vi "TCP Engine Device Name.vi"(8 "error in":errorcluster, 10 "Hardware Info":T1[](array[typedef]) {"Is Present?" items=["Initializing"=-2, "Unknown"=-1, "Not Present"=0, "Present"=1]}, 11 "JSON String":string) -> (0 "error out":errorcluster, 3 "Engine Name":string[](array[string]))   [LabVIEW 2024, in "TCP Engine.lvlib"]
doc: "This purpose of this VI is to get all engine names from JSON Commands. \n\n\n\nAll Rights Reserved © 2017 SyncSols"
uses:
  TCP Engine.lvlib
  Main Engine/Controls/Main Engine Hardware Info Data Cluster.ctl
  Host-DQMH/Configuration/All Interface Data.ctl
  Host-DQMH/Configuration/DO Channel's.ctl
  Host-DQMH/Configuration/Analog Input Single Channel Data--Cluster.ctl
  Host-DQMH/Configuration/Config-Channel Type.ctl
  Host-DQMH/Configuration/Channel Sub-Type.ctl
  Analog Output/Controls/AO Timing Cluster.ctl
  Async Serial/Controls/Async Serial Configuration Cluster.ctl
  Async Serial/Controls/Async Frame Info Cluster.ctl
  Async Serial/Controls/Async Message Info Cluster.ctl
  Async Serial/Controls/Async Update Cluster.ctl
  Ethernet/Controls/Ethernet Configuration Cluster.ctl
  Ethernet/Controls/Ethernet Frame Info Cluster.ctl
  Ethernet/Controls/Ethernet Message Info Cluster.ctl
  Ethernet/Controls/Ethernet Dynamic Data Cluster.ctl
  Ethernet/Controls/Ethernet Update Cluster.ctl
  <vilib>/Utility/error.llb/Error Cluster From Error Code.vi
  <userlib>/_OpenG.lib/array/array.llb/Remove Duplicates from 1D Array (String)__ogtk.vi
  <vilib>/ErrorRing/Error Ring.xnode
  <vilib>/regexp/Match Regular Expression.xnode
  <userlib>/_OpenG.lib/array/array.llb/openg_array.lvlib
  <userlib>/_OpenG.lib/string/string.llb/openg_string.lvlib
  Host-DQMH/Configuration/Configuration.lvlib
panel:
  out "concatenated string":string
  out "Data":string
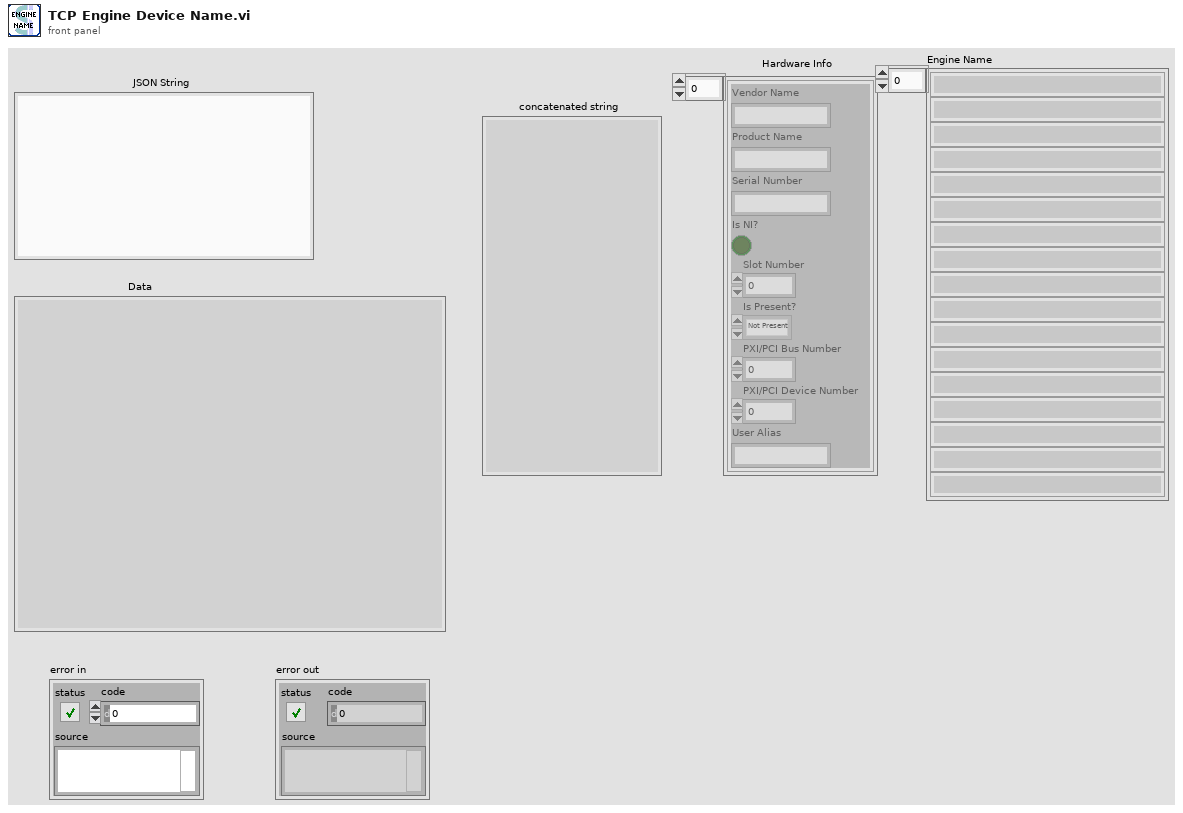
[diagram p1: front panel]
types:
  T1 = typedef "Main Engine Hardware Info Data Cluster.ctl" = cluster{"Vendor Name":string, "Product Name":string, "Serial Number":string, "Is NI?":bool, "Slot Number":i32, "Is Present?":i32, "PXI/PCI Bus Number":u32, "PXI/PCI Device Number":u32, "User Alias":string}
  T2 = typedef "Async Serial Configuration Cluster.ctl" = cluster{"Port":string, "Minor Frame Freq":u16, "Minor Frame Count":u16, "Frame Info":T3[], "Sensor Type":u16, "OIM Address":u16}
  T3 = typedef "Async Frame Info Cluster.ctl" = cluster{"Frame ID":u16, "Message Info":T4[]}
  T4 = typedef "Async Message Info Cluster.ctl" = cluster{"Message":u8[], "Message Name":string}
  T5 = typedef "Async Update Cluster.ctl" = cluster{"Port":string, "Message Info":T4[]}
  T6 = typedef "Ethernet Configuration Cluster.ctl" = cluster{"Mode":u8, "Local IP":string, "Local Port":u16, "Frame Info":T7[], "Minor Frame Freq":u8}
  T7 = typedef "Ethernet Frame Info Cluster.ctl" = cluster{"Frame ID":u16, "Message Info":T8[]}
  T8 = typedef "Ethernet Message Info Cluster.ctl" = cluster{"Message":u8[], "Message Name":string, "Dynamic":u8, "DynData":T9[], "Client IP":string, "Client Port":u16}
  T9 = typedef "Ethernet Dynamic Data Cluster.ctl" = cluster{"Type":string, "Start Byte":u8, "End Byte":u8, "Data":u32[][], "File Name":string, "Column":i32}
  T10 = typedef "Ethernet Update Cluster.ctl" = cluster{"IP":string, "Message Info":T4[], "Port":u16}
  T11 = typedef "Configuration.lvlib/All Interface Data.ctl" = cluster{"DI Config Data":T12, "DO Config Data":T12, "AI Config Data's":cluster{"Module Name":string, "AI Channel's Data":T13[], "Analog Input Timing":T16}[]}
  T12 = typedef "Configuration.lvlib/DO Channel's.ctl" = cluster{"Channel Name":string, "Identification Name":string, "Data":u8[], "Enabled?":bool}[]
  T13 = typedef "Configuration.lvlib/Analog Input Single Channel Data--Cluster.ctl" = cluster{"Channel Name":string, "Identification Name":string, "Channel Type":T14, "Sub-Type":T15, "Data":string, "Enabled?":bool}
  T14 = typedef "Configuration.lvlib/Config-Channel Type.ctl" = enum16{"Voltage", "Current", "Thermocouple", "Acclerometer"}
  T15 = typedef "Configuration.lvlib/Channel Sub-Type.ctl" = enum16{"None", "Pressure", "Force"}
  T16 = typedef "AO Timing Cluster.ctl" = cluster{"samples per channel":i32, "sample mode":i32, "Sampling Rate":dbl}
  T17 = cluster{"Module Name":string, "AI Channel's Data":T13[], "Analog Input Timing":T16}[]
  T18 = cluster{"Module Name":string, "AI Channel's Data":T13[], "Analog Input Timing":T16}
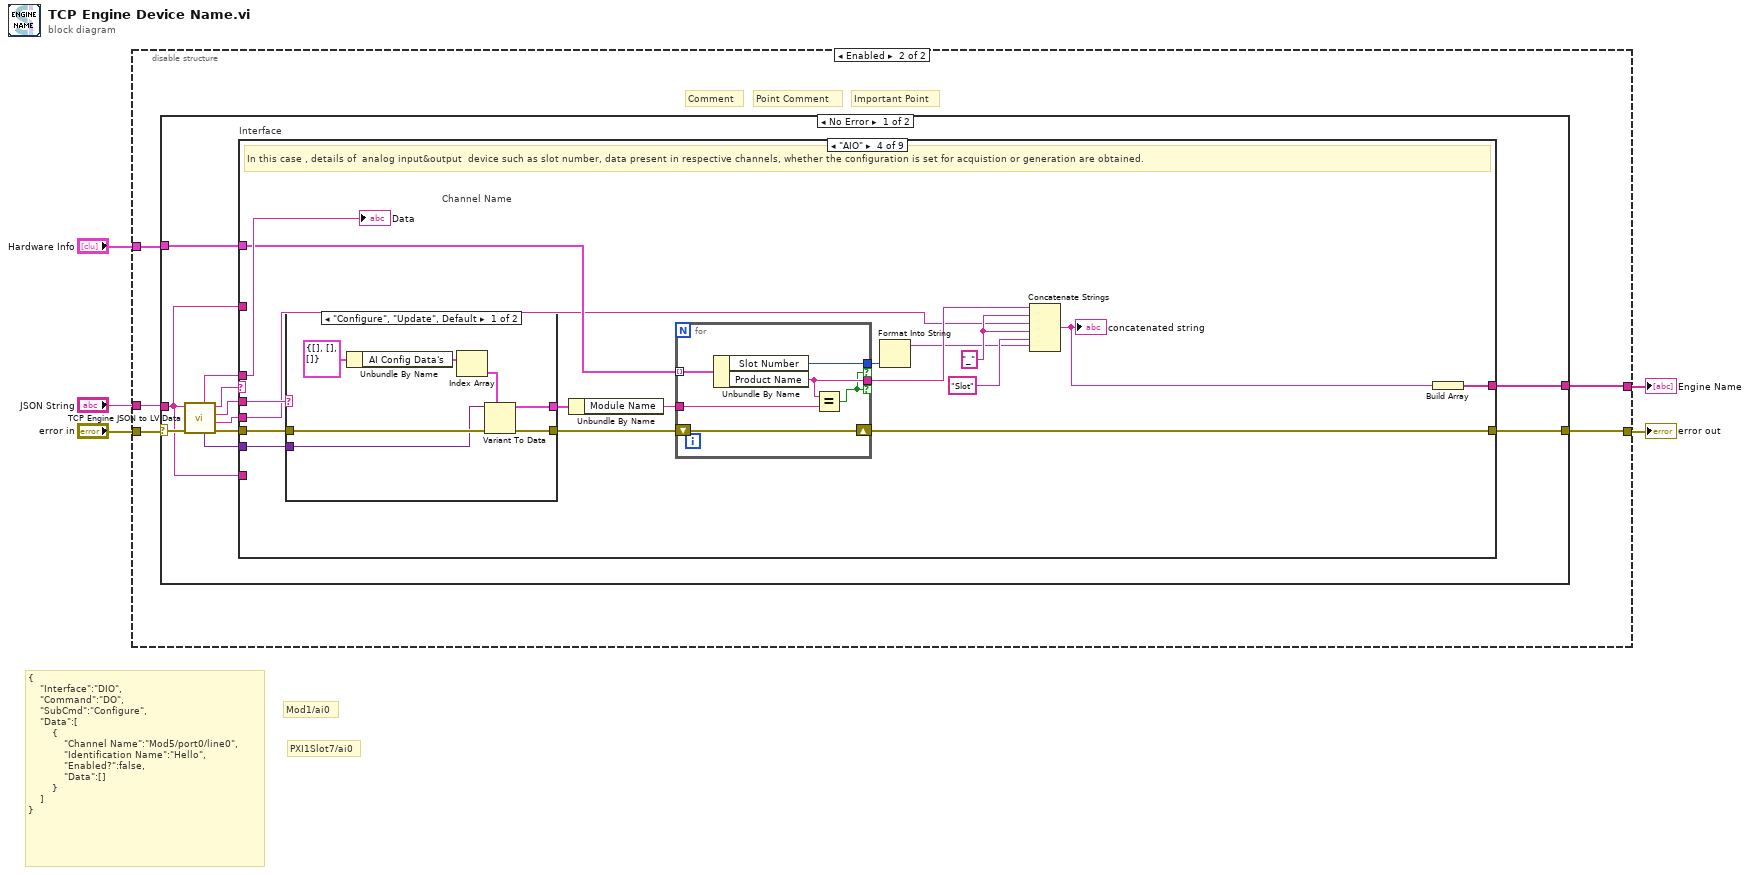
[diagram p0: block diagram]
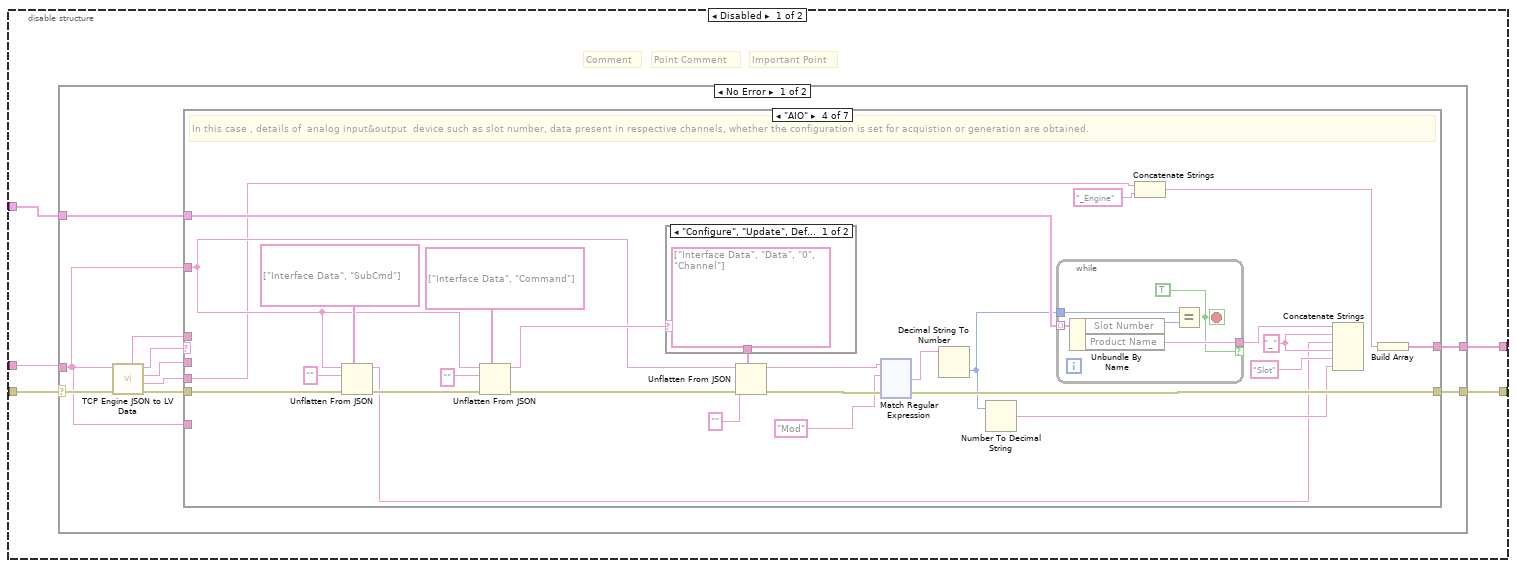
[diagram p2: hidden frame]
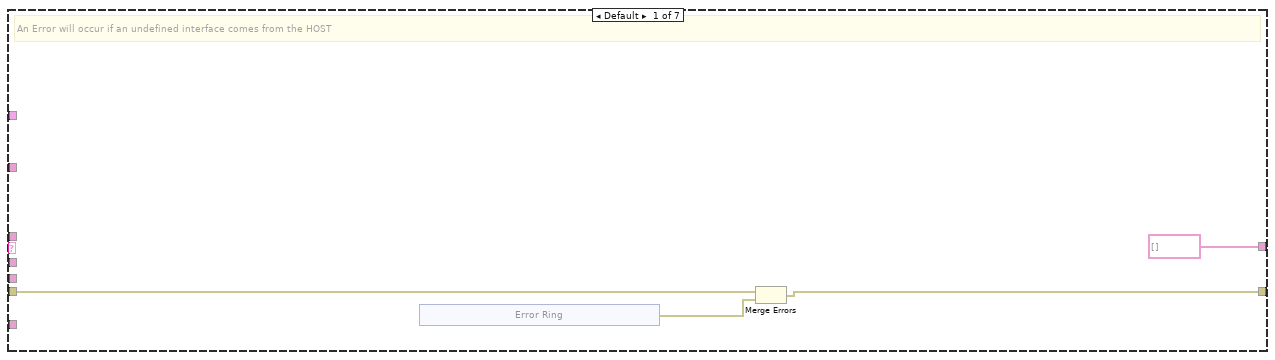
[diagram p3: hidden frame]
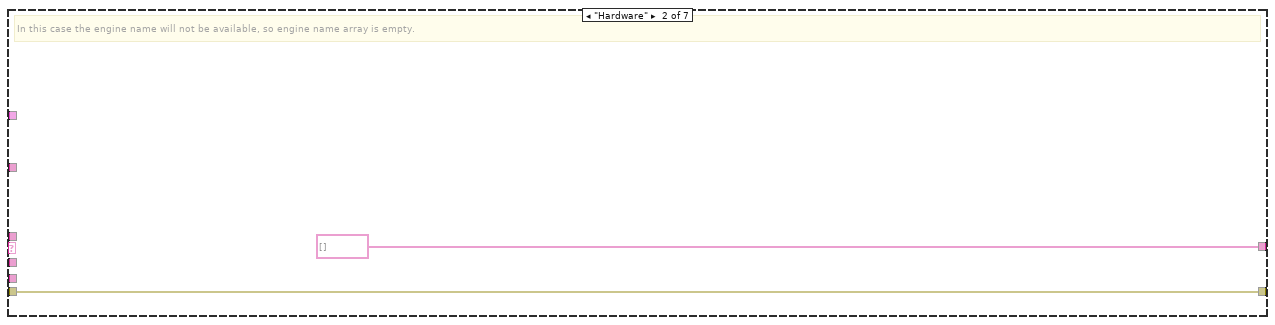
[diagram p4: hidden frame]
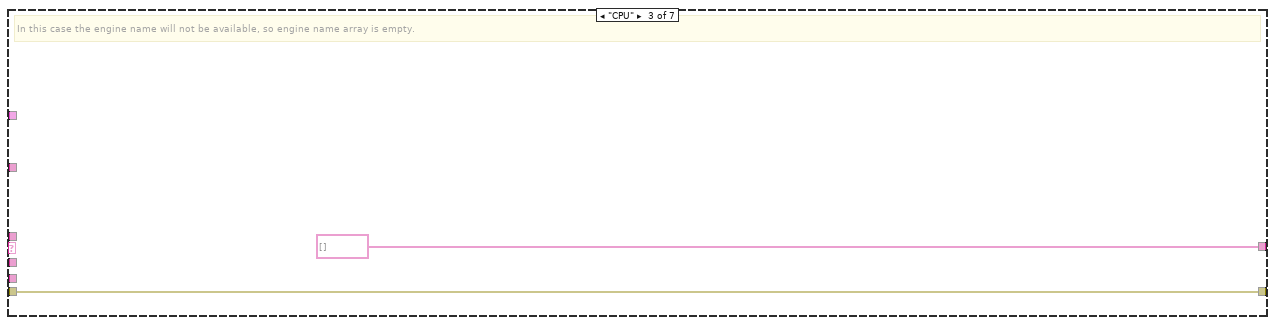
[diagram p5: hidden frame]
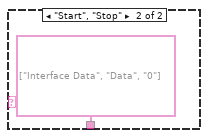
[diagram p6: hidden frame]
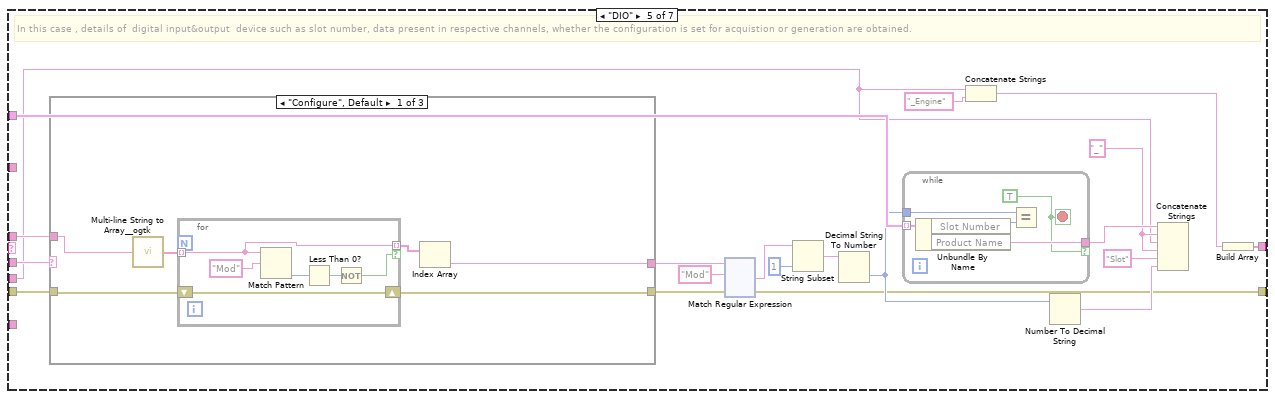
[diagram p7: hidden frame]
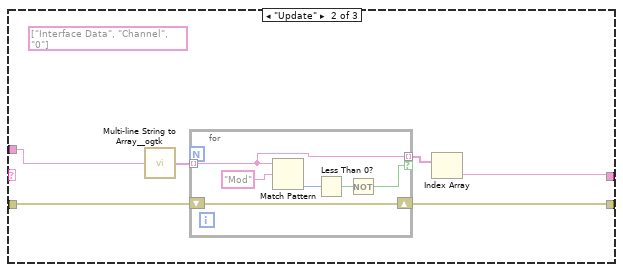
[diagram p8: hidden frame]
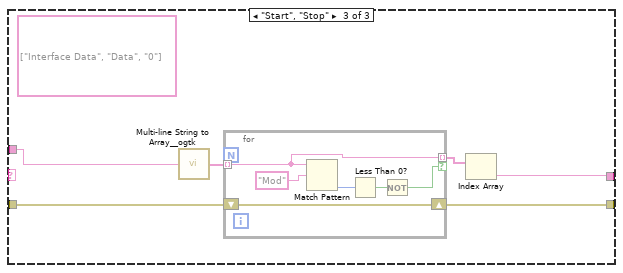
[diagram p9: hidden frame]
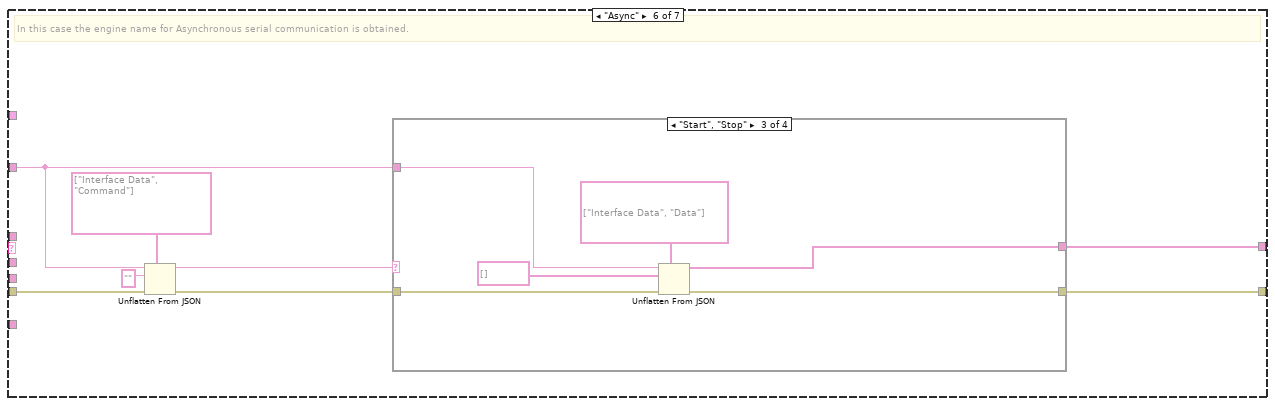
[diagram p10: hidden frame]
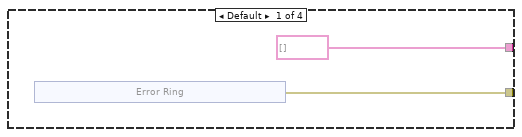
[diagram p11: hidden frame]
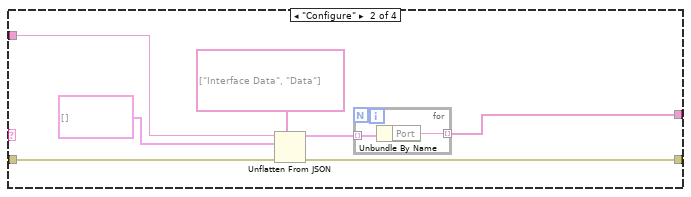
[diagram p12: hidden frame]
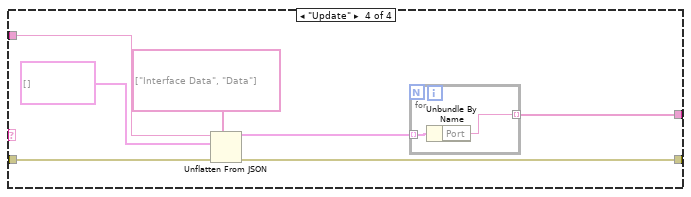
[diagram p13: hidden frame]
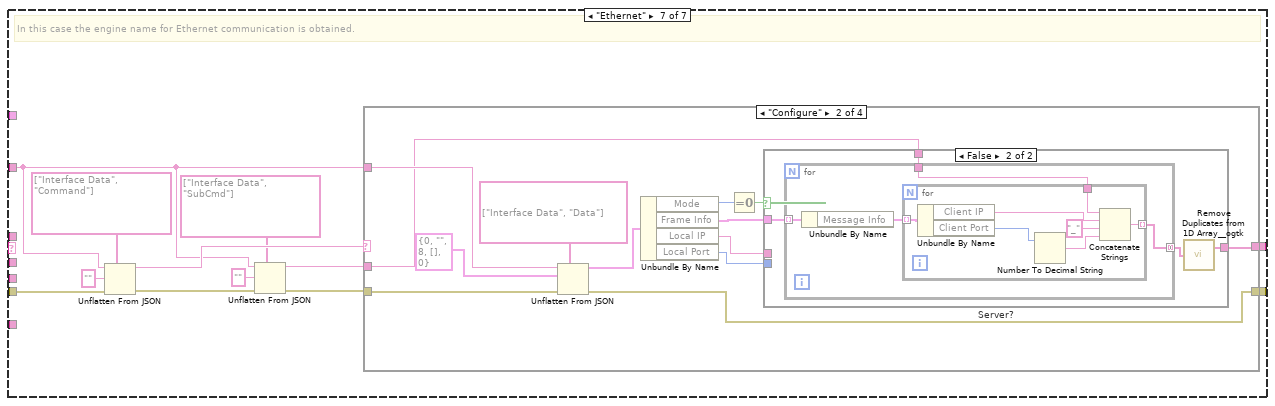
[diagram p14: hidden frame]
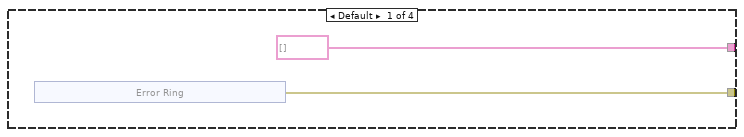
[diagram p15: hidden frame]
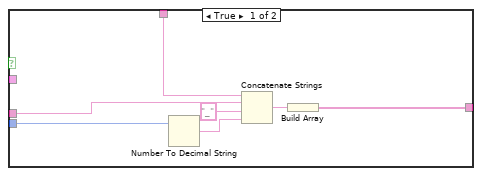
[diagram p16: hidden frame]
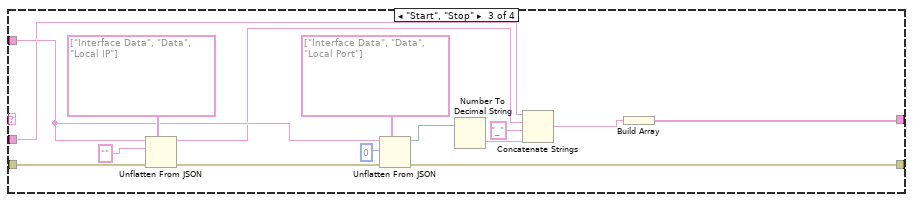
[diagram p17: hidden frame]
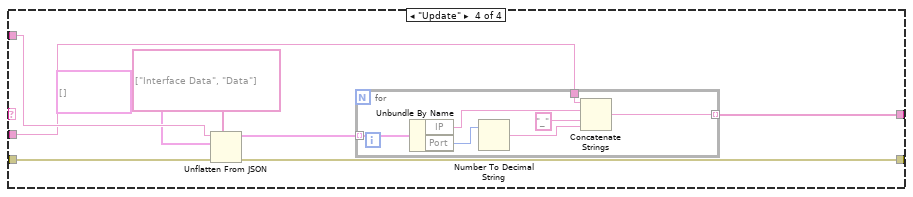
[diagram p18: hidden frame]
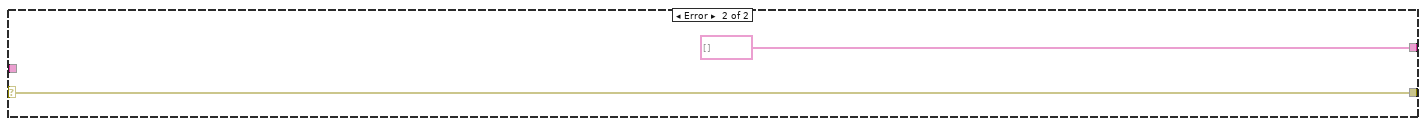
[diagram p19: hidden frame]
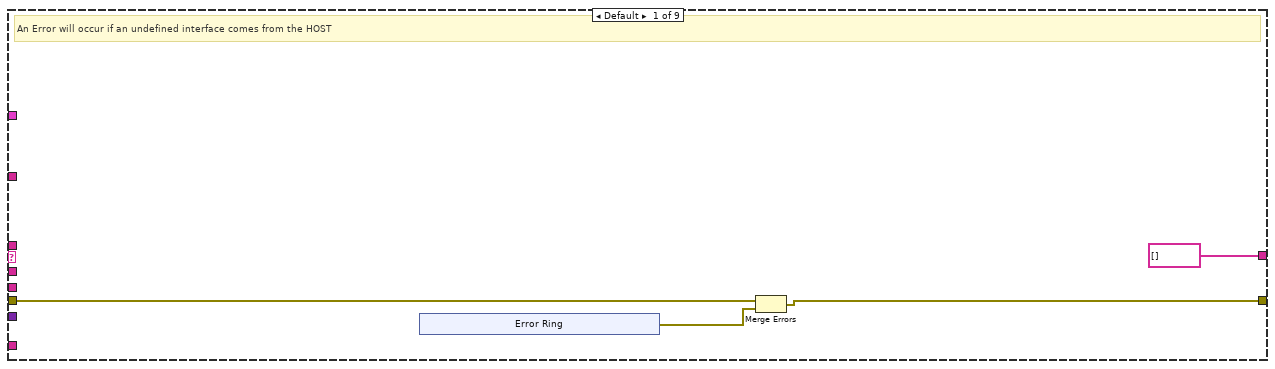
[diagram p20: hidden frame]
diagram:
  # "{\n    \"Interface\":\"DIO\",\n    \"Command\":\"DO\",\n    \"SubCmd\":\"Configure\",\n    \"Data\":[\n        {\n            \"Channel Name\":\"Mod5/port0/line0\",\n            \"Identification Name\":\"Hello\",\n            \"Enabled?\":false,\n            \"Data\":[]\n        }\n    ]\n}"
  # "Mod1/ai0"
  # "PXI1Slot7/ai0"
  n1 = disable-structure shown="Enabled" {
    disable-tunnel: "error in" -> [w10 w490]
    disable-tunnel: "JSON String" -> [w9 w491]
    disable-tunnel: "Hardware Info" -> [w8 w492]
    disable-tunnel: [w7 w488] -> w2
    disable-tunnel: [w6 w489] -> w1
    frame Disabled {
      # "Important Point"
      # "Point Comment"
      # "Comment"
      n2 = case shown="No Error" w10 {
        selector: w10 -> [w17 w487]
        tunnel: [w20 w487] -> w6
        tunnel: w9 -> [w15 _]
        tunnel: w8 -> [w19 _]
        tunnel: [w18 string[] [] ("Product Name")] -> w7
        frame No Error {
          n3 = call "TCP Engine JSON to LV Data.vi"("error in"=w17, "Cmd String"=w15) -> ("error out"=w16:errorcluster, "SubCmd"=w11:string, "Command"=w12:string, "Interface"=w14:string, "Data"=w13:string)  [unwired: 4 in, 1 out]
          n4 = case shown="\"AIO\"" w14 {
            tunnel: w15 -> [_ _ _ w37 _ w364 w403]
            tunnel: w16 -> [w21 w30 w32 w50 w198 w365 w409]
            tunnel: [w22 w30 w32 w56 w190 w370 w413] -> w20
            tunnel: w19 -> [_ _ _ w53 w204 _ _]
            tunnel: [string[] [] ("Product Name") string[] [] ("Product Name") string[] [] ("Product Name") w42 w200 w369 w412] -> w18
            tunnel: w15 -> [_ _ _ _ _ _ _]
            tunnel: w13 -> [_ _ _ _ w197 _ _]
            tunnel: w12 -> [_ _ _ _ w188 _ _]
            tunnel: w11 -> [_ _ _ w35 w187 _ _]
            frame Default {
              # "An Error will occur if an undefined interface comes from the HOST"
              n5 = xnode "Error Ring"() -> ("error out"=w24:errorcluster)
              n6 = Merge Errors(w21, w24) -> (w22:errorcluster)
            }
            frame "Hardware" {
              # "In this case the engine name will not be available, so engine name array is empty."
            }
            frame "CPU" {
              # "In this case the engine name will not be available, so engine name array is empty."
            }
            frame "AIO" {
              w41 = "_" ("string")
              # "In this case , details of  analog input&output  device such as slot number, data present in respective channels, whether the configuration is set for acquistion or generation are obtained."
              n7 = Unflatten From JSON(path=string[] ["Interface Data", "SubCmd"], JSON string=w37, type and defaults="", error in (no error)=w50) -> (value=w38:string, error out=w47:errorcluster)  [unwired: 3 in]
              n8 = Unflatten From JSON(path=string[] ["Interface Data", "Command"], JSON string=w37, type and defaults="", error in (no error)=w47) -> (value=w43:string, error out=w46:errorcluster)  [unwired: 3 in]
              n9 = case shown="\"Configure\", \"Update\", Default" w43 {
                tunnel: [string[] ["Interface Data", "Data", "0", "Channel"] ("path") string[] ["Interface Data", "Data", "0"] ("path")] -> w60
                frame "Configure", "Update", Default {
                }
                frame "Start", "Stop" {
                }
              }
              n10 = Unflatten From JSON(path=w60, JSON string=w37, type and defaults="", error in (no error)=w46) -> (value=w58:string, error out=w57:errorcluster)  [unwired: 3 in]
              n11 = xnode "Match Regular Expression"("input string"=w58, "regular expression"="Mod", "error in"=w57) -> ("after match"=w54:string, "error out"=w56:errorcluster)  [unwired: 3 in, 3 out]
              n12 = Decimal String To Number(string=w54) -> (number=w40:i32)  [unwired: 2 in, 1 out]
              n13 = Number To Decimal String(number=w40) -> (decimal integer string=w39:string)  [unwired: 1 in]
              n14 = while {
                tunnel: w53 -> [w184] mode=indexing
                tunnel: w40 -> [w182]
                tunnel: [w181] -> w52 if=w180
                stop <- w180 stop-if-true
                w180 = TRUE
                n15 = Unbundle By Name(w184) -> ("Slot Number"=w183:i32, "Product Name"=w181:string)
                n16 = Equal?(x=w182, y=w183) -> ()  [unwired: 1 out]
              }
              n17 = Concatenate Strings(w35, "_Engine" ("string")) -> (w34:string)
              n18 = Concatenate Strings(w52, w41, w38, w41, "Slot" ("string"), w39) -> ()  [unwired: 1 out]
              n19 = Build Array(w34) -> (w42:string[])
            }
            frame "DIO" {
              w201 = "_" ("string")
              # "In this case , details of  digital input&output  device such as slot number, data present in respective channels, whether the configuration is set for acquistion or generation are obtained."
              n20 = case shown="\"Configure\", Default" w188 {
                tunnel: [w323 w335 w348] -> w191
                tunnel: w198 -> [w322 w336 w349]
                tunnel: w197 -> [w325 w337 w347]
                tunnel: [w324 w334 w346] -> w189
                frame "Configure", Default {
                  n21 = call <userlib>:"Multi-line String to Array__ogtk.vi"("string"=w325) -> ("lines"=w327:string[])
                  n22 = for {
                    tunnel: w327 -> [w329] mode=indexing
                    tunnel: [w329] -> w326 mode=indexing if=w330
                    shift-right: [w328] -> w323
                    shift-left: w322 -> [w328]
                    n23 = Match Pattern(string=w329, regular expression="Mod") -> (offset past match=w332:i32)  [unwired: 1 in, 3 out]
                    n24 = Less Than 0?(x=w332) -> (x < 0?=w331:bool)
                    n25 = Not(x=w331) -> (.not. x?=w330:bool)
                  }
                  n26 = Index Array(array=w326) -> (element=w324:string)  [unwired: 1 in]
                }
                frame "Update" {
                  (unwired) string[] ["Interface Data", "Channel", "0"] ("path")
                  n27 = call <userlib>:"Multi-line String to Array__ogtk.vi"("string"=w337) -> ("lines"=w339:string[])
                  n28 = for {
                    tunnel: w339 -> [w341] mode=indexing
                    tunnel: [w341] -> w338 mode=indexing if=w342
                    shift-right: [w340] -> w335
                    shift-left: w336 -> [w340]
                    n29 = Match Pattern(string=w341, regular expression="Mod") -> (offset past match=w344:i32)  [unwired: 1 in, 3 out]
                    n30 = Less Than 0?(x=w344) -> (x < 0?=w343:bool)
                    n31 = Not(x=w343) -> (.not. x?=w342:bool)
                  }
                  n32 = Index Array(array=w338) -> (element=w334:string)  [unwired: 1 in]
                }
                frame "Start", "Stop" {
                  (unwired) string[] ["Interface Data", "Data", "0"] ("path")
                  n33 = call <userlib>:"Multi-line String to Array__ogtk.vi"("string"=w347) -> ("lines"=w351:string[])
                  n34 = for {
                    tunnel: w351 -> [w353] mode=indexing
                    tunnel: [w353] -> w350 mode=indexing if=w354
                    shift-right: [w352] -> w348
                    shift-left: w349 -> [w352]
                    n35 = Match Pattern(string=w353, regular expression="Mod") -> (offset past match=w356:i32)  [unwired: 1 in, 3 out]
                    n36 = Less Than 0?(x=w356) -> (x < 0?=w355:bool)
                    n37 = Not(x=w355) -> (.not. x?=w354:bool)
                  }
                  n38 = Index Array(array=w350) -> (element=w346:string)  [unwired: 1 in]
                }
              }
              n39 = xnode "Match Regular Expression"("input string"=w189, "regular expression"="Mod", "error in"=w191) -> ("after match"=w195:string, "error out"=w190:errorcluster)  [unwired: 3 in, 3 out]
              n40 = String Subset(string=w195, length (rest)=1 ("length (rest)")) -> (substring=w193:string)  [unwired: 1 in]
              n41 = Decimal String To Number(string=w193) -> (number=w192:i32)  [unwired: 2 in, 1 out]
              n42 = while {
                tunnel: w204 -> [w362] mode=indexing
                tunnel: w192 -> [w360]
                tunnel: [w359] -> w203 if=w358
                stop <- w358 stop-if-true
                w358 = TRUE
                n43 = Unbundle By Name(w362) -> ("Slot Number"=w361:i32, "Product Name"=w359:string)
                n44 = Equal?(x=w360, y=w361) -> ()  [unwired: 1 out]
              }
              n45 = Concatenate Strings(w187, "_Engine" ("string")) -> (w185:string)
              n46 = Number To Decimal String(number=w192) -> (decimal integer string=w199:string)  [unwired: 1 in]
              n47 = Concatenate Strings(w203, w201, w187, w201, "Slot" ("string"), w199) -> ()  [unwired: 1 out]
              n48 = Build Array(w185) -> (w200:string[])
            }
            frame "Async" {
              # "In this case the engine name for Asynchronous serial communication is obtained."
              n49 = Unflatten From JSON(path=string[] ["Interface Data", "Command"], JSON string=w364, type and defaults="", error in (no error)=w365) -> (value=w363:string, error out=w366:errorcluster)  [unwired: 3 in]
              n50 = case shown="\"Start\", \"Stop\"" w363 {
                tunnel: [w372 w384 w392 w394] -> w370
                tunnel: [string[] [] ("Data") w380 w387 w395] -> w369
                tunnel: w366 -> [_ w379 w390 w398]
                tunnel: w364 -> [_ w378 w389 w393]
                frame Default {
                  n51 = xnode "Error Ring"() -> ("error out"=w372:errorcluster)
                }
                frame "Configure" {
                  n52 = Unflatten From JSON(path=string[] ["Interface Data", "Data"], JSON string=w378, type and defaults=T2[] [] ("Data"), error in (no error)=w379) -> (value=w381:T2[], error out=w384:errorcluster)  [unwired: 3 in]
                  n53 = for {
                    tunnel: [w386] -> w380 mode=indexing
                    tunnel: w381 -> [w385] mode=indexing
                    n54 = Unbundle By Name(w385) -> ("Port"=w386:string)
                  }
                }
                frame "Start", "Stop" {
                  n55 = Unflatten From JSON(path=string[] ["Interface Data", "Data"], JSON string=w389, type and defaults=string[] [] ("Data"), error in (no error)=w390) -> (value=w387:string[], error out=w392:errorcluster)  [unwired: 3 in]
                }
                frame "Update" {
                  n56 = Unflatten From JSON(path=string[] ["Interface Data", "Data"], JSON string=w393, type and defaults=T5[] [] ("Array"), error in (no error)=w398) -> (value=w396:T5[], error out=w394:errorcluster)  [unwired: 3 in]
                  n57 = for {
                    tunnel: w396 -> [w401] mode=indexing
                    tunnel: [w400] -> w395 mode=indexing
                    n58 = Unbundle By Name(w401) -> ("Port"=w400:string)
                  }
                }
              }
            }
            frame "Ethernet" {
              # "In this case the engine name for Ethernet communication is obtained."
              n59 = Unflatten From JSON(path=string[] ["Interface Data", "Command"], JSON string=w403, type and defaults="", error in (no error)=w409) -> (value=w408:string, error out=w406:errorcluster)  [unwired: 3 in]
              n60 = Unflatten From JSON(path=string[] ["Interface Data", "SubCmd"], JSON string=w403, type and defaults="", error in (no error)=w406) -> (value=w404:string, error out=w407:errorcluster)  [unwired: 3 in]
              n61 = case shown="\"Configure\"" w408 {
                tunnel: [w415 w424 w464 w476] -> w413
                tunnel: [string[] [] ("Data") w426 w467 w472] -> w412
                tunnel: w407 -> [_ w432 w469 w477]
                tunnel: w403 -> [_ w431 w463 w475]
                tunnel: w404 -> [_ w425 w456 w471]
                frame Default {
                  n62 = xnode "Error Ring"() -> ("error out"=w415:errorcluster)
                }
                frame "Configure" {
                  n63 = Unflatten From JSON(path=string[] ["Interface Data", "Data"], JSON string=w431, type and defaults=T6 {"Mode"=0, "Local IP"="", "Local Port"=8, "Frame Info"=[], "Minor Frame Freq"=0} ("Ethernet Configuration"), error in (no error)=w432) -> (value=w429:T6, error out=w424:errorcluster)  [unwired: 3 in]
                  n64 = Unbundle By Name(w429) -> ("Mode"=w423:u8, "Frame Info"=w421:T7[], "Local IP"=w427:string, "Local Port"=w428:u16)
                  n65 = Equal To 0?(x=w423) -> (x = 0?=w422:bool)
                  n66 = case "Server?" shown="False" w422 {
                    tunnel: w428 -> [w440 _]
                    tunnel: w427 -> [w439 _]
                    tunnel: [w436 w441] -> w426
                    tunnel: w425 -> [w434 w444]
                    tunnel: w421 -> [_ w443]
                    frame True {
                      n67 = Number To Decimal String(number=w440) -> (decimal integer string=w438:string)  [unwired: 1 in]
                      n68 = Concatenate Strings(w434, w439, "_" ("string"), w438) -> (w437:string)
                      n69 = Build Array(w437) -> (w436:string[])
                    }
                    frame False {
                      n70 = for {
                        tunnel: [w445] -> w442 mode=concatenating
                        tunnel: w444 -> [w448]
                        tunnel: w443 -> [w447] mode=indexing
                        n71 = Unbundle By Name(w447) -> ("Message Info"=w446:T8[])
                        n72 = for {
                          tunnel: w448 -> [w453]
                          tunnel: w446 -> [w452] mode=indexing
                          tunnel: [w449] -> w445 mode=indexing
                          n73 = Unbundle By Name(w452) -> ("Client IP"=w451:string, "Client Port"=w450:u16)
                          n74 = Number To Decimal String(number=w450) -> (decimal integer string=w455:string)  [unwired: 1 in]
                          n75 = Concatenate Strings(w453, w451, "_" ("string"), w455) -> (w449:string)
                        }
                      }
                      n76 = call-poly <userlib>:"Remove Duplicates from 1D Array__ogtk.vi"("Input Array"=w442) -> ("Output Array"=w441:string[])  [unwired: 1 out]
                    }
                  }
                }
                frame "Start", "Stop" {
                  n77 = Unflatten From JSON(path=string[] ["Interface Data", "Data", "Local IP"], JSON string=w463, type and defaults="", error in (no error)=w469) -> (value=w461:string, error out=w465:errorcluster)  [unwired: 3 in]
                  n78 = Unflatten From JSON(path=string[] ["Interface Data", "Data", "Local Port"], JSON string=w463, type and defaults=u16 0, error in (no error)=w465) -> (value=w457:u16, error out=w464:errorcluster)  [unwired: 3 in]
                  n79 = Number To Decimal String(number=w457) -> (decimal integer string=w458:string)  [unwired: 1 in]
                  n80 = Concatenate Strings(w456, w461, "_" ("string"), w458) -> (w460:string)
                  n81 = Build Array(w460) -> (w467:string[])
                }
                frame "Update" {
                  n82 = Unflatten From JSON(path=string[] ["Interface Data", "Data"], JSON string=w475, type and defaults=T10[] [] ("value"), error in (no error)=w477) -> (value=w473:T10[], error out=w476:errorcluster)  [unwired: 3 in]
                  n83 = for {
                    tunnel: w473 -> [w485] mode=indexing
                    tunnel: [w480] -> w472 mode=indexing
                    tunnel: w471 -> [w479]
                    n84 = Unbundle By Name(w485) -> ("IP"=w482:string, "Port"=w484:u16)
                    n85 = Number To Decimal String(number=w484) -> (decimal integer string=w483:string)  [unwired: 1 in]
                    n86 = Concatenate Strings(w479, w482, "_" ("string"), w483) -> (w480:string)
                  }
                }
              }
            }
          }
        }
        frame Error {
        }
      }
    }
    frame Enabled {
      # "Important Point"
      # "Point Comment"
      # "Comment"
      n87 = case shown="No Error" w490 {
        selector: w490 -> [w500 w685]
        tunnel: [w503 w685] -> w489
        tunnel: w491 -> [w498 _]
        tunnel: w492 -> [w502 _]
        tunnel: [w501 string[] [] ("Product Name")] -> w488
        frame No Error {
          n88 = call "TCP Engine JSON to LV Data.vi"("error in"=w500, "Cmd String"=w498) -> ("error out"=w499:errorcluster, "SubCmd"=w494:string, "Command"=w495:string, "Interface"=w497:string, 4:"Data"=w493:variant, 5:"Data"=w496:string)  [unwired: 4 in]
          n89 = case "Interface" shown="\"AIO\"" w497 {
            tunnel: w498 -> [_ _ _ _ _ w560 w599 _ _]
            tunnel: w499 -> [w504 w513 w515 w527 w554 w561 w605 w682 w683]
            tunnel: [w505 w513 w515 w517 w554 w566 w609 w682 w683] -> w503
            tunnel: w502 -> [_ _ _ w530 _ _ _ _ _]
            tunnel: [string[] [] ("Product Name") string[] [] ("Product Name") string[] [] ("Product Name") w519 w558 w565 w608 _ _] -> w501
            tunnel: w498 -> [_ _ _ _ _ _ _ _ _]
            tunnel: w496 -> [_ _ _ w531 _ _ _ _ _]
            tunnel: w495 -> [_ _ _ w528 _ _ _ _ _]
            tunnel: w494 -> [_ _ _ w523 w557 _ _ _ _]
            tunnel: w493 -> [_ _ _ w526 _ _ _ _ _]
            frame Default {
              # "An Error will occur if an undefined interface comes from the HOST"
              n90 = xnode "Error Ring"() -> ("error out"=w507:errorcluster)
              n91 = Merge Errors(w504, w507) -> (w505:errorcluster)
            }
            frame "Hardware" {
              # "In this case the engine name will not be available, so engine name array is empty."
            }
            frame "CPU" {
              # "In this case the engine name will not be available, so engine name array is empty."
            }
            frame "AIO" {
              w532 = "_" ("string")
              # "Channel Name"
              # "In this case , details of  analog input&output  device such as slot number, data present in respective channels, whether the configuration is set for acquistion or generation are obtained."
              n92 = case shown="\"Configure\", \"Update\", Default" w528 {
                tunnel: w527 -> [w546 w550]
                tunnel: w526 -> [w545 w549]
                tunnel: [w544 w548] -> w518
                tunnel: [w540 w547] -> w525
                frame "Configure", "Update", Default {
                  n93 = Unbundle By Name(T11 {"DI Config Data"=[], "DO Config Data"=[], "AI Config Data's"=[]} ("Interface Data")) -> ("AI Config Data's"=w543:T17)
                  n94 = Index Array(array=w543) -> (element=w541:T18)  [unwired: 1 in]
                  n95 = Variant To Data(error in=w546, type=w541, Variant=w545) -> (data=w540:T18, error out=w544:errorcluster)
                }
                frame "Start", "Stop" {
                  n96 = Unbundle By Name(T11 {"DI Config Data"=[], "DO Config Data"=[], "AI Config Data's"=[]} ("Interface Data")) -> ("AI Config Data's"=w553:T17)
                  n97 = Index Array(array=w553) -> (element=w551:T18)  [unwired: 1 in]
                  n98 = Variant To Data(error in=w550, type=w551, Variant=w549) -> (data=w547:T18, error out=w548:errorcluster)
                }
              }
              n99 = Unbundle By Name(w525) -> ("Module Name"=w524:string)
              n100 = for {
                tunnel: [w538] -> w529 if=w535
                tunnel: w530 -> [w539] mode=indexing
                tunnel: w524 -> [w537]
                tunnel: [w536] -> w522 if=w535
                shift-right: [w534] -> w517
                shift-left: w518 -> [w534]
                n101 = Unbundle By Name(w539) -> ("Slot Number"=w536:i32, "Product Name"=w538:string)
                n102 = Equal?(x=w538, y=w537) -> (x = y?=w535:bool)
              }
              n103 = Format Into String(w522) -> (resulting string=w521:string)  [unwired: 3 in, 1 out]
              n104 = Concatenate Strings(w529, w532, w523, w532, "Slot" ("string"), w521) -> (w520:string)
              "concatenated string" <- w520
              n105 = Build Array(w520) -> (w519:string[])
              "Data" <- w531
            }
            frame "DIO" {
              # "In this case , details of  digital input&output  device such as slot number, data present in respective channels, whether the configuration is set for acquistion or generation are obtained."
              n106 = Concatenate Strings(w557, "_Engine" ("string")) -> (w555:string)
              n107 = Build Array(w555) -> (w558:string[])
            }
            frame "Async" {
              # "In this case the engine name for Asynchronous serial communication is obtained."
              n108 = Unflatten From JSON(path=string[] ["Interface Data", "Command"], JSON string=w560, type and defaults="", error in (no error)=w561) -> (value=w559:string, error out=w562:errorcluster)  [unwired: 3 in]
              n109 = case shown="\"Start\", \"Stop\"" w559 {
                tunnel: [w568 w580 w588 w590] -> w566
                tunnel: [string[] [] ("Data") w576 w583 w591] -> w565
                tunnel: w562 -> [_ w575 w586 w594]
                tunnel: w560 -> [_ w574 w585 w589]
                frame Default {
                  n110 = xnode "Error Ring"() -> ("error out"=w568:errorcluster)
                }
                frame "Configure" {
                  n111 = Unflatten From JSON(path=string[] ["Interface Data", "Data"], JSON string=w574, type and defaults=T2[] [] ("Data"), error in (no error)=w575) -> (value=w577:T2[], error out=w580:errorcluster)  [unwired: 3 in]
                  n112 = for {
                    tunnel: [w582] -> w576 mode=indexing
                    tunnel: w577 -> [w581] mode=indexing
                    n113 = Unbundle By Name(w581) -> ("Port"=w582:string)
                  }
                }
                frame "Start", "Stop" {
                  n114 = Unflatten From JSON(path=string[] ["Interface Data", "Data"], JSON string=w585, type and defaults=string[] [] ("Data"), error in (no error)=w586) -> (value=w583:string[], error out=w588:errorcluster)  [unwired: 3 in]
                }
                frame "Update" {
                  n115 = Unflatten From JSON(path=string[] ["Interface Data", "Data"], JSON string=w589, type and defaults=T5[] [] ("Array"), error in (no error)=w594) -> (value=w592:T5[], error out=w590:errorcluster)  [unwired: 3 in]
                  n116 = for {
                    tunnel: w592 -> [w597] mode=indexing
                    tunnel: [w596] -> w591 mode=indexing
                    n117 = Unbundle By Name(w597) -> ("Port"=w596:string)
                  }
                }
              }
            }
            frame "Ethernet" {
              # "In this case the engine name for Ethernet communication is obtained."
              n118 = Unflatten From JSON(path=string[] ["Interface Data", "Command"], JSON string=w599, type and defaults="", error in (no error)=w605) -> (value=w604:string, error out=w602:errorcluster)  [unwired: 3 in]
              n119 = Unflatten From JSON(path=string[] ["Interface Data", "SubCmd"], JSON string=w599, type and defaults="", error in (no error)=w602) -> (value=w600:string, error out=w603:errorcluster)  [unwired: 3 in]
              n120 = case shown="\"Configure\"" w604 {
                tunnel: [w611 w620 w660 w672] -> w609
                tunnel: [string[] [] ("Data") w622 w663 w668] -> w608
                tunnel: w603 -> [_ w628 w665 w673]
                tunnel: w599 -> [_ w627 w659 w671]
                tunnel: w600 -> [_ w621 w652 w667]
                frame Default {
                  n121 = xnode "Error Ring"() -> ("error out"=w611:errorcluster)
                }
                frame "Configure" {
                  n122 = Unflatten From JSON(path=string[] ["Interface Data", "Data"], JSON string=w627, type and defaults=T6 {"Mode"=0, "Local IP"="", "Local Port"=8, "Frame Info"=[], "Minor Frame Freq"=0} ("Ethernet Configuration"), error in (no error)=w628) -> (value=w625:T6, error out=w620:errorcluster)  [unwired: 3 in]
                  n123 = Unbundle By Name(w625) -> ("Mode"=w619:u8, "Frame Info"=w617:T7[], "Local IP"=w623:string, "Local Port"=w624:u16)
                  n124 = Equal To 0?(x=w619) -> (x = 0?=w618:bool)
                  n125 = case "Server?" shown="False" w618 {
                    tunnel: w624 -> [w636 _]
                    tunnel: w623 -> [w635 _]
                    tunnel: [w632 w637] -> w622
                    tunnel: w621 -> [w630 w640]
                    tunnel: w617 -> [_ w639]
                    frame True {
                      n126 = Number To Decimal String(number=w636) -> (decimal integer string=w634:string)  [unwired: 1 in]
                      n127 = Concatenate Strings(w630, w635, "_" ("string"), w634) -> (w633:string)
                      n128 = Build Array(w633) -> (w632:string[])
                    }
                    frame False {
                      n129 = for {
                        tunnel: [w641] -> w638 mode=concatenating
                        tunnel: w640 -> [w644]
                        tunnel: w639 -> [w643] mode=indexing
                        n130 = Unbundle By Name(w643) -> ("Message Info"=w642:T8[])
                        n131 = for {
                          tunnel: w644 -> [w649]
                          tunnel: w642 -> [w648] mode=indexing
                          tunnel: [w645] -> w641 mode=indexing
                          n132 = Unbundle By Name(w648) -> ("Client IP"=w647:string, "Client Port"=w646:u16)
                          n133 = Number To Decimal String(number=w646) -> (decimal integer string=w651:string)  [unwired: 1 in]
                          n134 = Concatenate Strings(w649, w647, "_" ("string"), w651) -> (w645:string)
                        }
                      }
                      n135 = call-poly <userlib>:"Remove Duplicates from 1D Array__ogtk.vi"("Input Array"=w638) -> ("Output Array"=w637:string[])  [unwired: 1 out]
                    }
                  }
                }
                frame "Start", "Stop" {
                  n136 = Unflatten From JSON(path=string[] ["Interface Data", "Data", "Local IP"], JSON string=w659, type and defaults="", error in (no error)=w665) -> (value=w657:string, error out=w661:errorcluster)  [unwired: 3 in]
                  n137 = Unflatten From JSON(path=string[] ["Interface Data", "Data", "Local Port"], JSON string=w659, type and defaults=u16 0, error in (no error)=w661) -> (value=w653:u16, error out=w660:errorcluster)  [unwired: 3 in]
                  n138 = Number To Decimal String(number=w653) -> (decimal integer string=w654:string)  [unwired: 1 in]
                  n139 = Concatenate Strings(w652, w657, "_" ("string"), w654) -> (w656:string)
                  n140 = Build Array(w656) -> (w663:string[])
                }
                frame "Update" {
                  n141 = Unflatten From JSON(path=string[] ["Interface Data", "Data"], JSON string=w671, type and defaults=T10[] [] ("value"), error in (no error)=w673) -> (value=w669:T10[], error out=w672:errorcluster)  [unwired: 3 in]
                  n142 = for {
                    tunnel: w669 -> [w681] mode=indexing
                    tunnel: [w676] -> w668 mode=indexing
                    tunnel: w667 -> [w675]
                    n143 = Unbundle By Name(w681) -> ("IP"=w678:string, "Port"=w680:u16)
                    n144 = Number To Decimal String(number=w680) -> (decimal integer string=w679:string)  [unwired: 1 in]
                    n145 = Concatenate Strings(w675, w678, "_" ("string"), w679) -> (w676:string)
                  }
                }
              }
            }
            frame "Exit" {
            }
            frame "General" {
            }
          }
        }
        frame Error {
        }
      }
    }
  }
  "error out" <- w1
  "Engine Name" <- w2
